vi "SwerveDriveDoesDevRefExist.vi"(0 "SwerveDriveDevRefArray":T1[](array[typedef]), 7 "SwerveDriveDevRef":T1={"DevStatus"={"status"=FALSE, "code"=0, "source"=""}, "TurnMotors[]"=[], "Square Inputs"=FALSE, "Max Output"=1.0, "DriveMotors[]"=[], "WheelOffset[]"=[], "SwerveSensors[]"=[], "RobotSize"={"Width"=[], "Length"=[], "Center"=[]}}) -> (4 "index":i32, 8 "exists":bool)   [LabVIEW 2019, in "Swerve Drive.lvlib"]
doc: "This is used to find the index of a DevRef within an array of DevRefs."
uses:
  Swerve Drive.lvlib
  SwerveDriveDevRef.ctl
  <vilib>/Rock Robotics/WPI/MotorControl/WPI_MotorControlDeviceRef.ctl
  <vilib>/Rock Robotics/WPI/MotorControl/WPI_MotorControlType.ctl
  <vilib>/Rock Robotics/SystemInterfaces/DIO/FPGA_DIOPWMChannel.ctl
  <vilib>/Rock Robotics/WPI/PWM/WPI_PWMDeadband.ctl
  <vilib>/Rock Robotics/SystemInterfaces/DIO/FPGA_DIOChannel.ctl
  <vilib>/Rock Robotics/SystemInterfaces/AI/FPGA_AIChannel.ctl
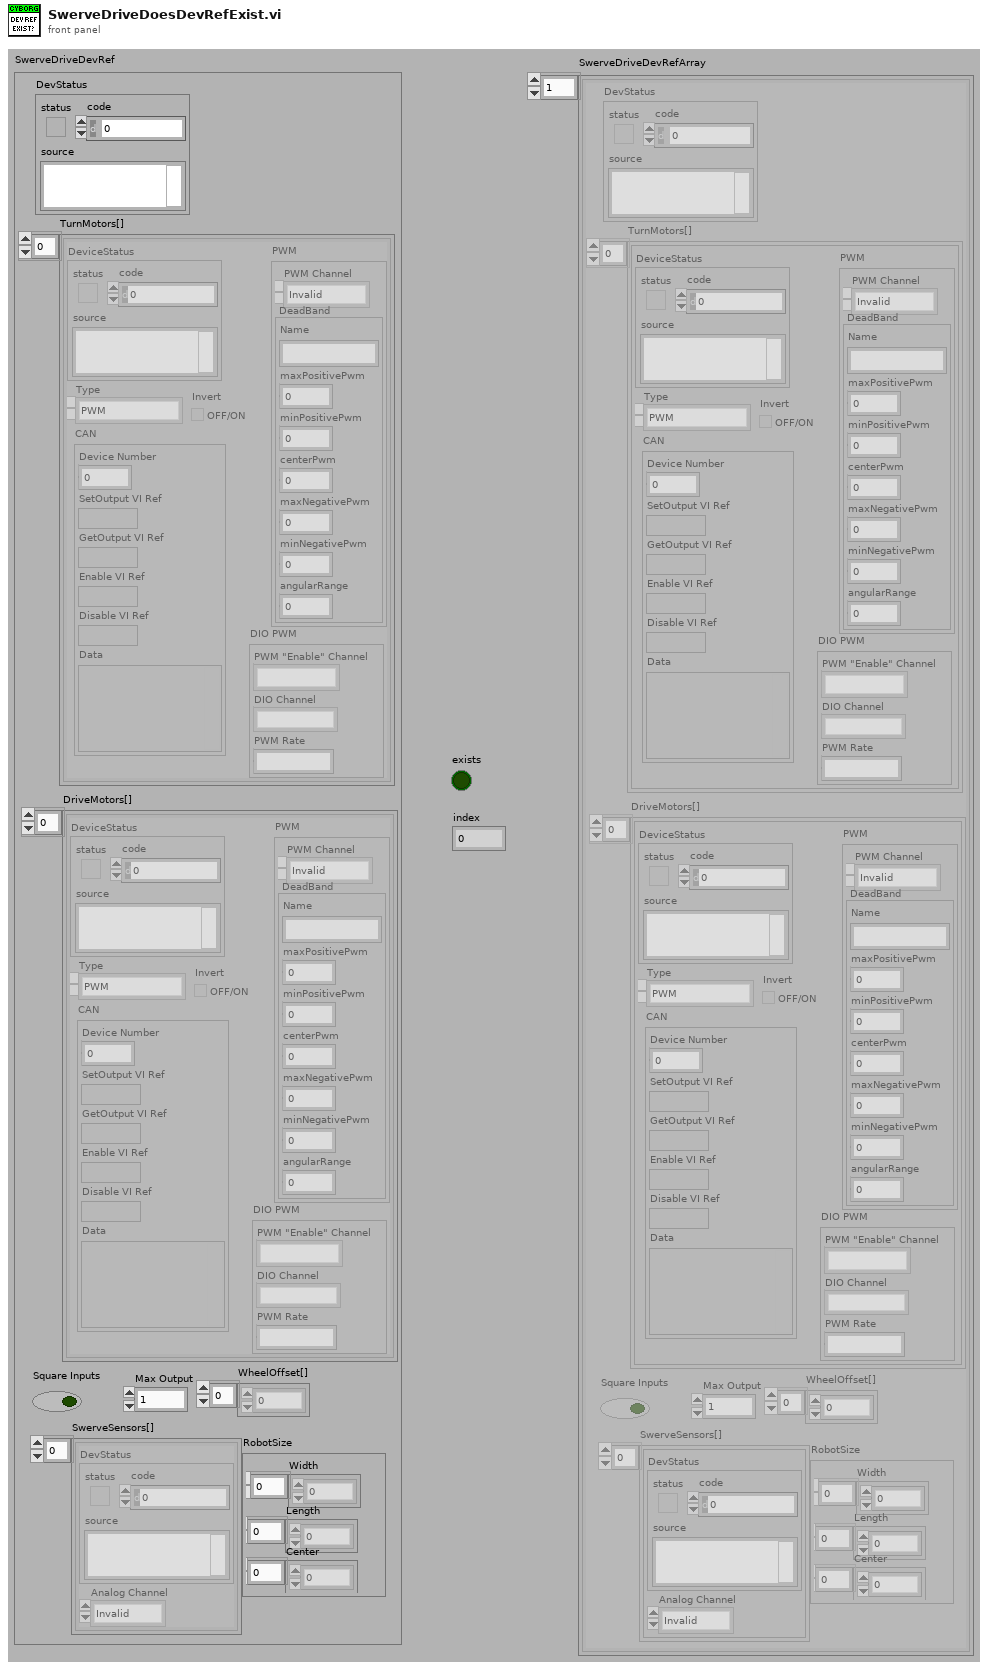
[diagram p1: front panel]
types:
  T1 = typedef "Swerve Drive.lvlib/SwerveDriveDevRef.ctl" = cluster{"DevStatus":errorcluster, "TurnMotors[]":T2[], "Square Inputs":bool, "Max Output":dbl, "DriveMotors[]":T2[], "WheelOffset[]":dbl[], "SwerveSensors[]":cluster{"DevStatus":errorcluster, "Analog Channel":T7}[], "RobotSize":cluster{"Width":dbl[], "Length":dbl[], "Center":dbl[]}}
  T2 = typedef "WPI_MotorControlDeviceRef.ctl" = cluster{"DeviceStatus":errorcluster, "Type":T3, "PWM":cluster{"PWM Channel":T4, "DeadBand":T5}, "CAN":cluster{"Device Number":u8, "SetOutput VI Ref":variant, "GetOutput VI Ref":variant, "Enable VI Ref":variant, "Disable VI Ref":variant, "Data":variant}, "Invert":bool, "DIO PWM":cluster{"PWM \"Enable\" Channel":T4, "DIOChannel":T6, "PWM Rate":dbl}}
  T3 = typedef "WPI_MotorControlType.ctl" = enum16{"PWM", "CAN", "DIO PWM"}
  T4 = typedef "FPGA_DIOPWMChannel.ctl" = enum8{"PWM 0", "PWM 1", "PWM 2", "PWM 3", "PWM 4", "PWM 5", "PWM 6", "PWM 7", "PWM 8", "PWM 9", "PWM MXP 0", "PWM MXP 1", "PWM MXP 2", "PWM MXP 3", "PWM MXP 4", "PWM MXP 5", "PWM MXP 6", "PWM MXP 7", "PWM MXP 8", "PWM MXP 9", "Invalid"}
  T5 = typedef "WPI_PWMDeadband.ctl" = cluster{"Name":string, "maxPositivePwm":i32, "minPositivePwm":i32, "centerPwm":i32, "maxNegativePwm":i32, "minNegativePwm":i32, "angularRange":u16}
  T6 = typedef "FPGA_DIOChannel.ctl" = enum8{"DIO 0", "DIO 1", "DIO 2", "DIO 3", "DIO 4", "DIO 5", "DIO 6", "DIO 7", "DIO 8", "DIO 9", "DIO MXP 0", "DIO MXP 1", "DIO MXP 2", "DIO MXP 3", "DIO MXP 4", "DIO MXP 5", "DIO MXP 6", "DIO MXP 7", "DIO MXP 8", "DIO MXP 9", "DIO MXP 10", "DIO MXP 11", "DIO MXP 12", "DIO MXP 13", "DIO MXP 14", "DIO MXP 15", "SPI Port CS1", "SPI Port CS2", "SPI Port CS3", "SPI Port MISO", "SPI Port MOSI", "Invalid"}
  T7 = typedef "FPGA_AIChannel.ctl" = enum8{"AI 0", "AI 1", "AI 2", "AI 3", "AI MXP 0", "AI MXP 1", "AI MXP 2", "AI MXP 3", "Invalid"}
  T8 = cluster{"[0]":T4, "[1]":T4, "[2]":T4, "[3]":T4, "[4]":T4, "[5]":T4, "[6]":T4, "[7]":T4, "[8]":T4}
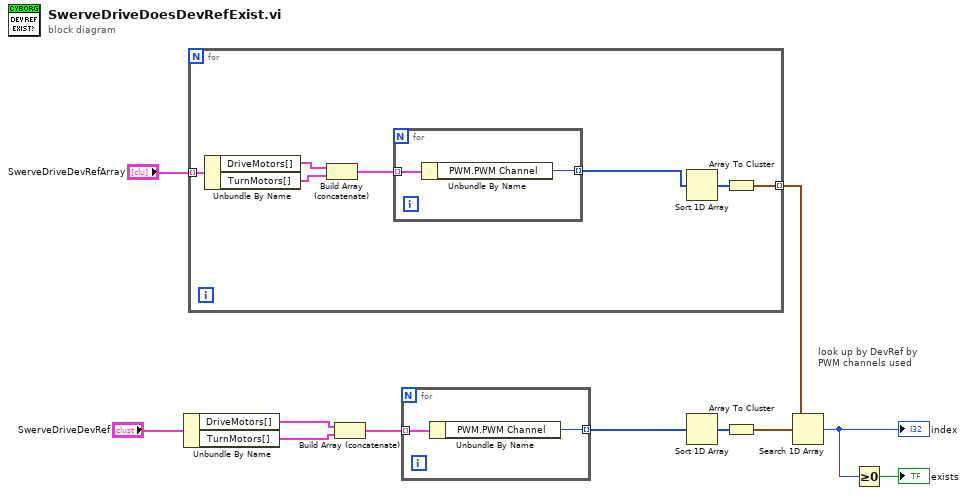
[diagram p0: block diagram]
diagram:
  # "look up by DevRef by PWM channels used"
  n1 = Unbundle By Name("SwerveDriveDevRef") -> ("DriveMotors[]"=w3:T2[], "TurnMotors[]"=w2:T2[])
  n2 = for {
    tunnel: [w17] -> w11 mode=indexing
    tunnel: "SwerveDriveDevRefArray" -> [w16] mode=indexing
    n3 = Unbundle By Name(w16) -> ("DriveMotors[]"=w13:T2[], "TurnMotors[]"=w14:T2[])
    n4 = Build Array (concatenate)(w13, w14) -> (w12:T2[])
    n5 = for {
      tunnel: w12 -> [w20] mode=indexing
      tunnel: [w19] -> w15 mode=indexing
      n6 = Unbundle By Name(w20) -> ("PWM.PWM Channel"=w19:T4)
    }
    n7 = Sort 1D Array(array=w15) -> (sorted array=w18:T4[])
    n8 = Array To Cluster(array=w18) -> (cluster=w17:T8)
  }
  n9 = Build Array (concatenate)(w3, w2) -> (w4:T2[])
  n10 = for {
    tunnel: w4 -> [w22] mode=indexing
    tunnel: [w21] -> w1 mode=indexing
    n11 = Unbundle By Name(w22) -> ("PWM.PWM Channel"=w21:T4)
  }
  n12 = Sort 1D Array(array=w1) -> (sorted array=w8:T4[])
  n13 = Array To Cluster(array=w8) -> (cluster=w7:T8)
  n14 = Search 1D Array(1D array=w11, element=w7) -> (index of element=w9:i32)  [unwired: 1 out]
  "index" <- w9
  n15 = Greater Or Equal To 0?(x=w9) -> (x >= 0?=→"exists":bool)
